vi "Read Min Max Waveform [MmW] Core.vi"(0 "IVI_Scope in":refnum<class "IVI_Scope.lvclass">, 1 "channel name (\"CHANNEL1\")":string="CHANNEL1", 2 "maximum time (5000ms)":i32=5000, 3 "waveform size (0)":i32=1000 caption="waveform size (1000)", 5 "error in (no error)":errorcluster) -> (11 "max waveform array":dbl[unit][](array[numeric]) format="%.3f", 13 "min waveform array":dbl[unit][](array[numeric]) format="%.3f", 14 "IVI_Scope out":refnum<class "IVI_Scope.lvclass">, 15 "actual points":i32, 16 "initial x":dbl[unit] format="%^.2e", 17 "x increment":dbl[unit] format="%^.2e", 19 "error out":errorcluster)   [LabVIEW 2016, in "IVI_Scope.lvlib" / "IVI_Scope.lvclass"]
doc: "This VI initiates an acquisition on all channels that you enable with the IviScope Configure Channel VI. If the channel you specify in the Channel Name parameter is not enabled for the acquisition, this VI returns the IVISCOPE_ERROR_CHANNEL_NOT_ENABLED (0xBFFA2001) error. It then waits for the acquisition to complete and returns the min/max waveforms for the channel you specify. If the oscilloscope did not complete the acquisition within the time period you specify with the Maximum Time parameter, the VI returns the IVISCOPE_ERROR_MAX_TIME_EXCEEDED (0xBFFA2003) error.\n\nYou call the IviScope Fetch Min Max Waveform [MmW] VI to obtain the waveforms for each of the remaining enabled channels without initiating another acquisition.\n\nNotes: \n\n(1) Use this VI to read waveforms when you set the acquisition type to IVISCOPE_VAL_PEAK_DETECT or IVISCOPE_VAL_ENVELOPE. If the acquisition type is not one of the listed types, the VI returns the IVISCOPE_ERROR_INVALID_ACQ_TYPE (0xBFFA2004) error.\n\n(2) After this VI executes, each element in the Min Waveform Array and Max Waveform Array parameters is either a voltage or a value indicating that the oscilloscope could not sample a voltage.\n\n(3) You configure the interpolation method the oscilloscope uses with the IviScope Is Invalid Waveform Element VI. If you disable interpolation, the oscilloscope does not interpolate points in the waveform. If the oscilloscope cannot sample a value for a point in the waveform, the driver sets the corresponding element in the Waveform Array to an IEEE defined NaN (Not a Number) value and the VI returns IVISCOPE_WARN_INVALID_WFM_ELEMENT (0x3FFA2001). \n\n(4) You can test a waveform value for an invalid value condition by calling the IviScope Is Invalid Waveform Element VI.\n\n(5) This VI performs interchangeability checking when the IviScope>>Inherent IVI Settings>>User Options>>Interchange Check property is set to TRUE. If the IviScope>>Inherent IVI Settings>>User Options>>Spy property is set to TRUE, you use the NI I/O Trace utility to view interchangeability warnings. You use the IviScope Get Next Interchange Warning VI to retrieve interchangeability warnings when the IviScope>>Inherent IVI Settings>>User Options>>Spy property is set to FALSE. For more information about interchangeability checking, refer to the help text for the IviScope>>Inherent IVI Settings>>User Options>>Interchange Check property.\n\n(6) The class driver returns simulated minimum and maximum waveforms when this VI is called and the IviScope>>Inherent IVI Settings>>User Options>>Simulate property is set to TRUE and the IviScope>>Inherent IVI Settings>>User Options>>Use Specific Simulation property is set to FALSE. For information on how to configure a simulated waveform, refer to the online help manual.\n\n(7) This VI is part of the IviScopeMinMaxWaveform [MmW] extension group."
uses:
  IVI_Scope.lvclass
  IVI_Scope.lvclass/IVI_Scope.ctl
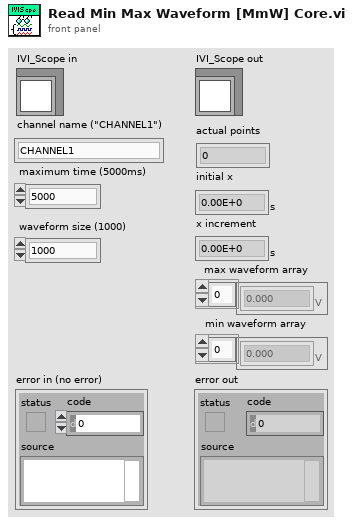
[diagram p1: front panel]
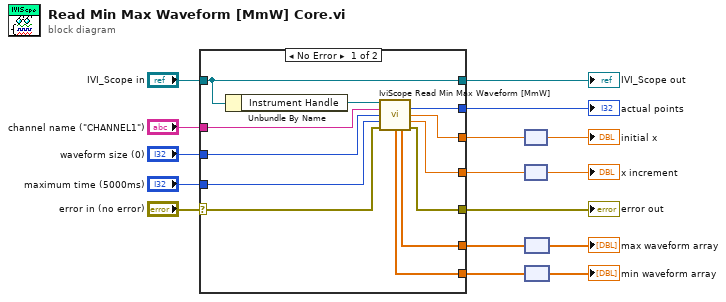
[diagram p0: block diagram]
diagram:
  n1 = case shown="No Error" "error in (no error)" {
    selector: "error in (no error)" -> [w26 w30]
    tunnel: [w25 w30] -> w15
    tunnel: [w28 w29] -> w13
    tunnel: "IVI_Scope in" -> [w28 w29]
    tunnel: "channel name (\"CHANNEL1\")" -> [w24 _]
    tunnel: "waveform size (0)" -> [w23 _]
    tunnel: "maximum time (5000ms)" -> [w22 _]
    tunnel: [w21 _] -> w9
    tunnel: [w20 _] -> w8
    tunnel: [w19 _] -> w6
    tunnel: [w18 _] -> w2
    tunnel: [w17 _] -> w4
    frame No Error {
      n2 = Unbundle By Name(w28) -> ("Instrument Handle"=w27:refnum<k15>)
      n3 = call <vilib>:"IviScope Read Min Max Waveform [MmW].vi"("instrument handle"=w27, "channel name (\"CHANNEL1\")"=w24, "waveform size (0)"=w23, "maximum time (5000ms)"=w22, "error in (no error)"=w26) -> ("actual points"=w21:i32, "initial x"=w20:dbl, "x increment"=w19:dbl, "min waveform array"=w18:dbl[], "max waveform array"=w17:dbl[], "error out"=w25:errorcluster)  [unwired: 4 in, 1 out]
    }
    frame Error {
    }
  }
  "error out" <- w15
  "IVI_Scope out" <- w13
  "actual points" <- w9
  n4 = node(w8) -> (→"initial x":dbl[unit])
  n5 = node(w6) -> (→"x increment":dbl[unit])
  n6 = node(w4) -> (→"max waveform array":dbl[unit][])
  n7 = node(w2) -> (→"min waveform array":dbl[unit][])
